vi "GUI_Plasma2_cap_pressure_cal.vi"() -> ()   [LabVIEW 2013]
uses:
  Shared/GUI_Template/GUI_master/tcp_new_data_event.ctl
  Shared/GUI_Template/GUI_master/tcp new data cluster.ctl
  <vilib>/Analysis/NI_AALBase.lvlib
  <vilib>/Analysis/NI_AALPro.lvlib
panel:
  in  "voltage::2":dbl=0.001 caption="voltage" min=0.0 max=30.0 format="%#.3f"
  in  "GUIdevice 2":string="P2-capHV"
  out "pressure::1":dbl=0.001 caption="Pressure" min=-100.0 max=500.0 format="%#.3f"
  in  "Tab Control":T1(tab)
  out "Pressure":dbl(graph)
  in  "points to save":T2(ring)
  in  "clear buffer":bool
  in  "send data":T2(ring)
  out "feed pressure":cluster{dbl[], dbl[]}(graph)
  out "cap pressure":cluster{dbl[], dbl[]}(graph)
  in  "combine plots":bool
  out "XY Graph 2":cluster{"ind":dbl[], "ini2":dbl[]}[](graph)=[{"ind"=[-2.02123979383, -1.9193278234999998, -1.81603094787, -1.7156190046100002, -1.6146447489499998, -1.51219345453, -1.4118886632300003, -1.3132607968099999, -1.20859797921, -1.10528298126, -0.99947359182, -0.89101754336, -0.7830056618400001, -0.6703321602099999, -0.560133506, -0.45195395803, -0.33700739742999997, -0.22552528281, -0.11709424518, -0.00137819706, 0.11140632129999999, 0.22448127726, 0.34074782323999997, 0.45065273575, 0.5650082886, 0.68208983815, 0.79504242345, 0.91265498684, 1.02879685929, 1.14707402107, 1.26927132994], "ini2"=[325.9, 334.1, 414.7, 495.2, 600.9, 746.4, 853.9, 1001.9, 1112.0, 1295.3, 1395.5, 1514.7, 1653.1, 1697.2, 1749.0, 1762.6, 1725.7, 1610.9, 1491.6, 1395.8, 1147.7, 1104.4, 888.0, 763.9, 613.5, 460.9, 375.1, 348.9, 338.1, 301.2, 290.0]}, {"ind"=[-2.02123979383, -2.02123979383, -2.02123979383, -1.9193278234999998, -1.9193278234999998, -1.9193278234999998, -1.81603094787, -1.81603094787, -1.81603094787, -1.7156190046100002, -1.7156190046100002, -1.7156190046100002, -1.6146447489499998, -1.6146447489499998, -1.6146447489499998, -1.51219345453, -1.51219345453, -1.51219345453, -1.4118886632300003, -1.4118886632300003, -1.4118886632300003, -1.3132607968099999, -1.3132607968099999, -1.3132607968099999, -1.20859797921, -1.20859797921, -1.20859797921, -1.10528298126, -1.10528298126, -1.10528298126, -0.99947359182, -0.99947359182, -0.99947359182, -0.89101754336, -0.89101754336, -0.89101754336, -0.7830056618400001, -0.7830056618400001, -0.7830056618400001, -0.6703321602099999, -0.6703321602099999, -0.6703321602099999, -0.560133506, -0.560133506, -0.560133506, -0.45195395803, -0.45195395803, -0.45195395803, -0.33700739742999997, -0.33700739742999997, -0.33700739742999997, -0.22552528281, -0.22552528281, -0.22552528281, -0.11709424518, -0.11709424518, -0.11709424518, -0.00137819706, -0.00137819706, -0.00137819706, 0.11140632129999999, 0.11140632129999999, 0.11140632129999999, 0.22448127726, 0.22448127726, 0.22448127726, 0.34074782323999997, 0.34074782323999997, 0.34074782323999997, 0.45065273575, 0.45065273575, 0.45065273575, 0.5650082886, 0.5650082886, 0.5650082886, 0.68208983815, 0.68208983815, 0.68208983815, 0.79504242345, 0.79504242345, 0.79504242345, 0.91265498684, 0.91265498684, 0.91265498684, 1.02879685929, 1.02879685929, 1.02879685929, 1.14707402107, 1.14707402107, 1.14707402107, 1.26927132994, 1.26927132994, 1.26927132994], "ini2"=[347.24088408040615, 304.5591159195938, nan, 345.14988687724906, 323.050113122751, nan, 451.6325210500327, 377.76747894996726, nan, 550.571071468372, 439.82892853162804, nan, 647.2044274341018, 554.5955725658981, nan, 805.5930926901291, 687.2069073098709, nan, 922.3502252248546, 785.4497747751453, nan, 1045.7974815779776, 958.0025184220223, nan, 1155.936823331284, 1068.063176668716, nan, 1360.6589235597473, 1229.9410764402526, nan, 1468.004789113854, 1322.995210886146, nan, 1570.967318321661, 1458.4326816783391, nan, 1710.4148225931904, 1595.7851774068095, nan, 1733.5311925974852, 1660.868807402515, nan, 1789.7376429798726, 1708.2623570201274, nan, 1800.3512325037946, 1724.8487674962053, nan, 1767.5623405408198, 1683.8376594591803, nan, 1653.6510883552169, 1568.1489116447833, nan, 1552.2083969246653, 1430.9916030753345, nan, 1464.0833963875716, 1327.5166036124283, nan, 1195.138966636675, 1100.2610333633252, nan, 1174.7928658001333, 1034.0071341998669, nan, 956.8896057310374, 819.1103942689626, nan, 863.6835991867734, 664.1164008132265, nan, 680.985389365238, 546.014610634762, nan, 522.2178422465906, 399.5821577534093, nan, 409.11127264109166, 341.0887273589084, nan, 373.0589642897943, 324.74103571020567, nan, 350.24221286806215, 325.9577871319379, nan, 316.5318839894733, 285.8681160105267, nan, 301.05541596785133, 278.94458403214867, nan]}] caption="output graph"
  out "slope":dbl
  out "intercept":dbl
  in  "GUIdevice 1":string="P2_PDR2000"
  in  "stop":bool
  out "tcp data event":T3
  out "error IO 2":errorcluster
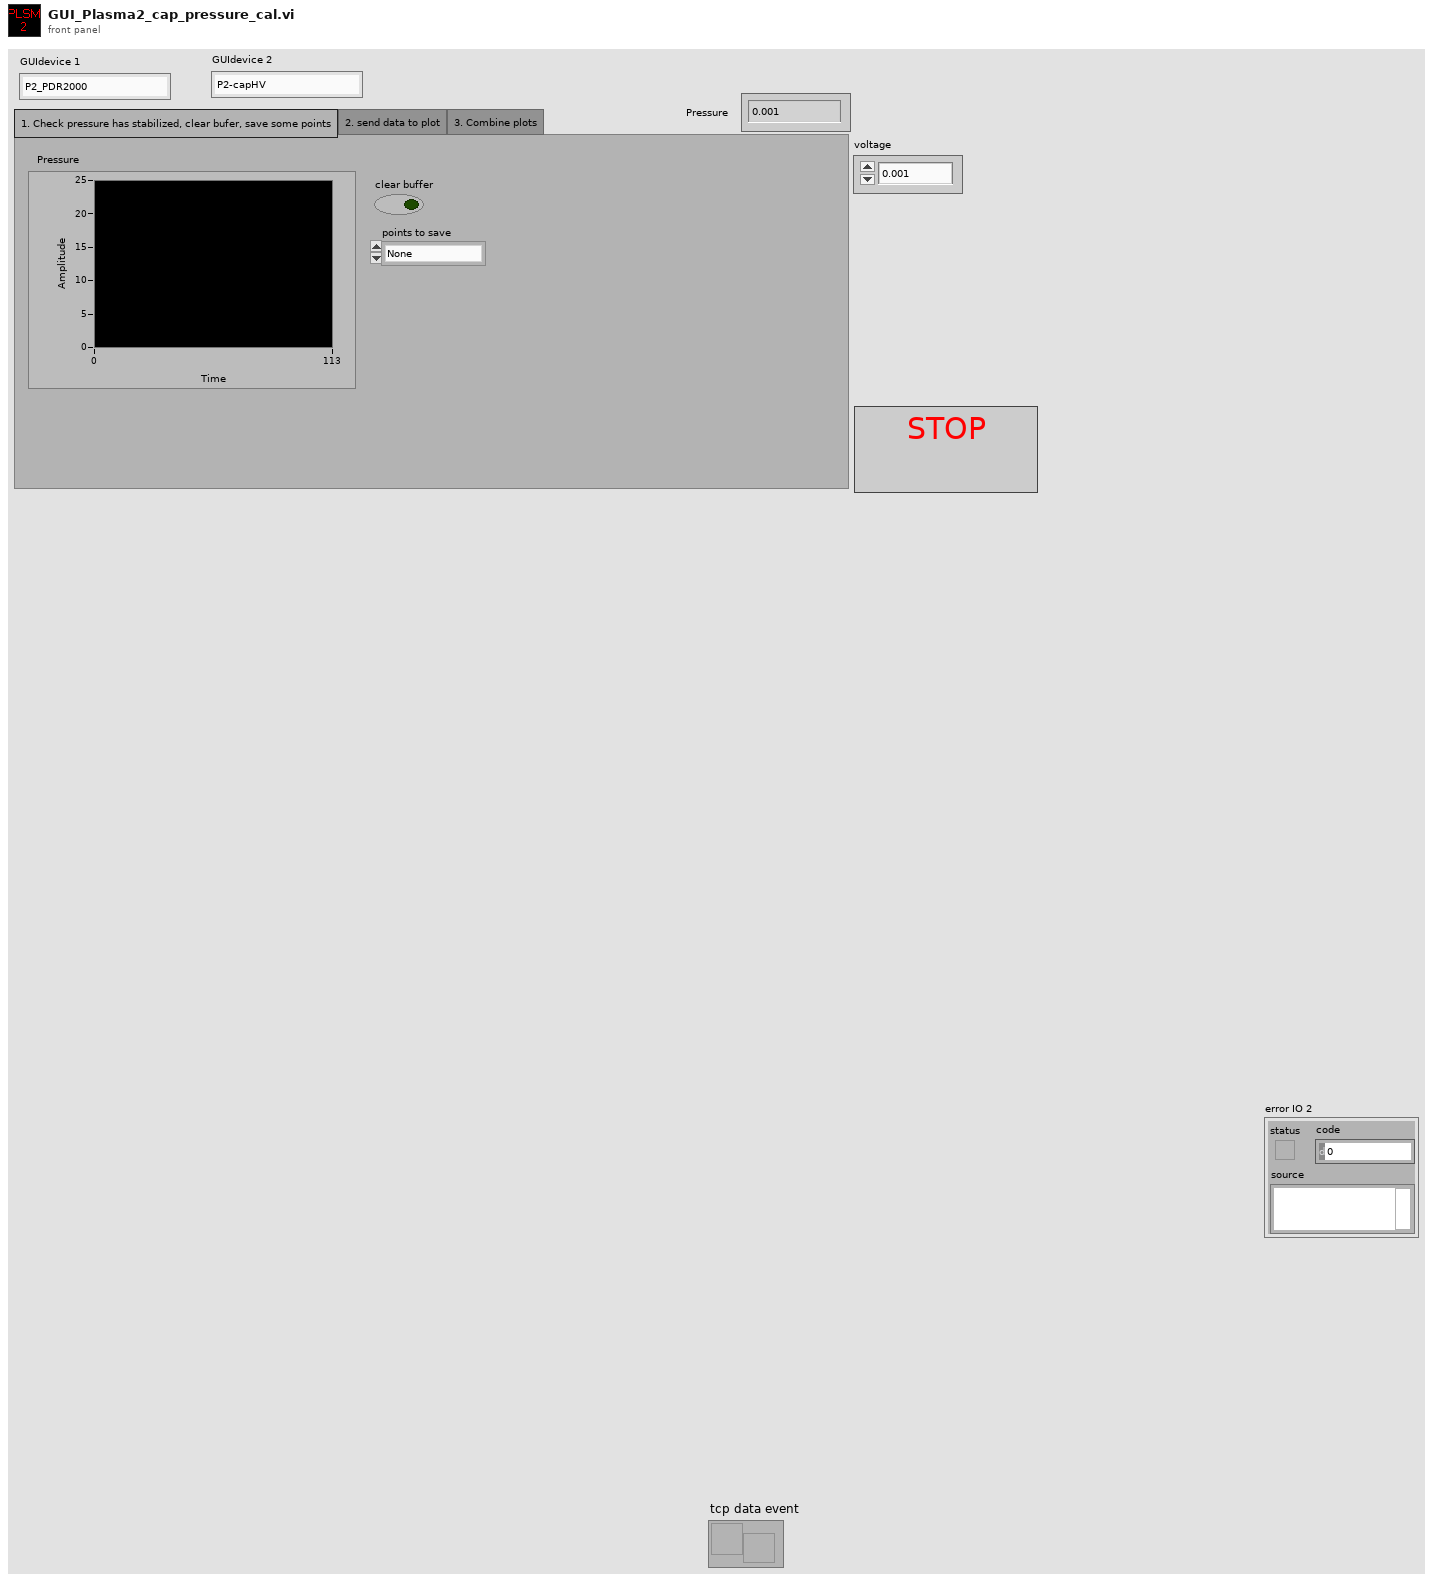
[diagram p1: front panel]
types:
  T1 = enum32{"1. Check pressure has stabilized, clear bufer, save some points", "2. send data to plot", "3. Combine plots"}
  T2 = enum16{"None", "Capillary pressure", "Feed pressure"}
  T3 = typedef "tcp_new_data_event.ctl" = refnum<user-event>
  T4 = typedef "tcp new data cluster.ctl" = cluster{"EventEnum":enum16{"new data", "connection status update"}, "Device name":string}
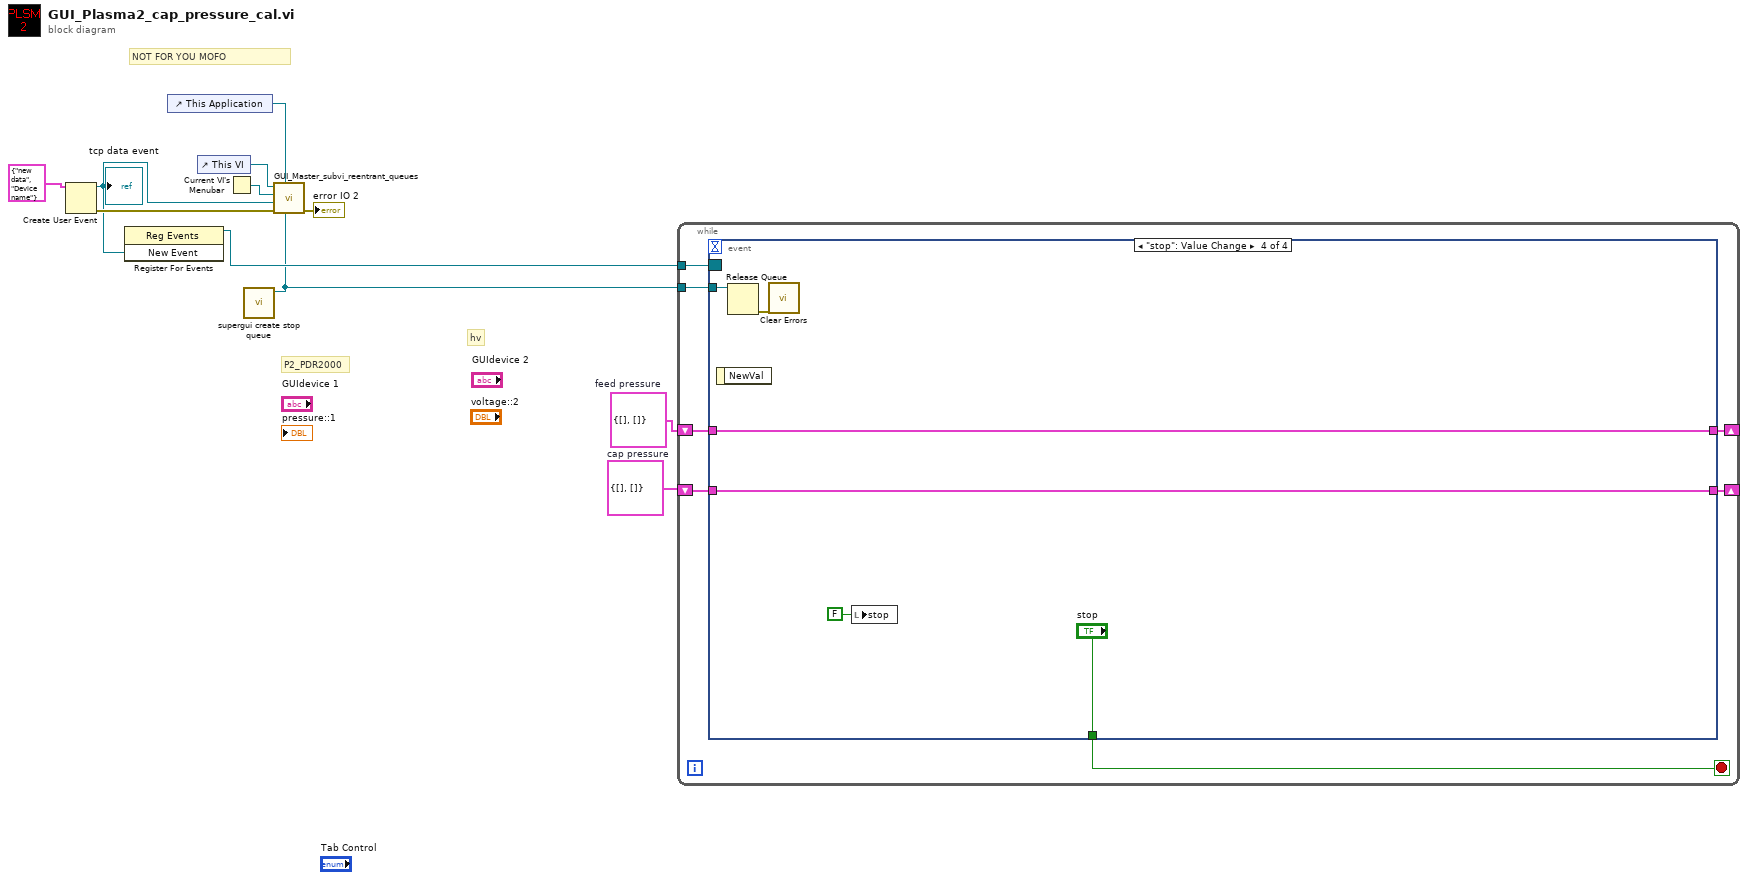
[diagram p0: block diagram]
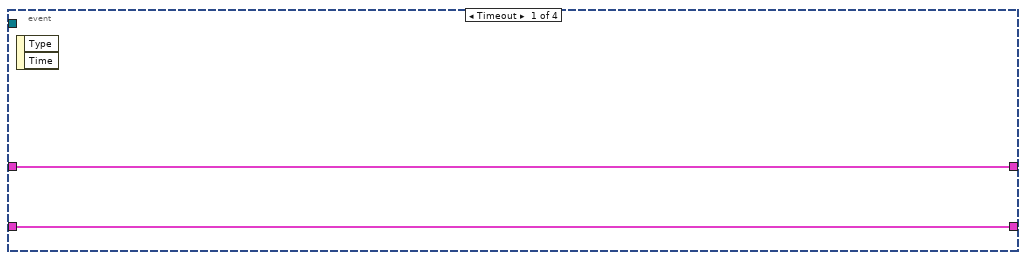
[diagram p2: hidden frame]
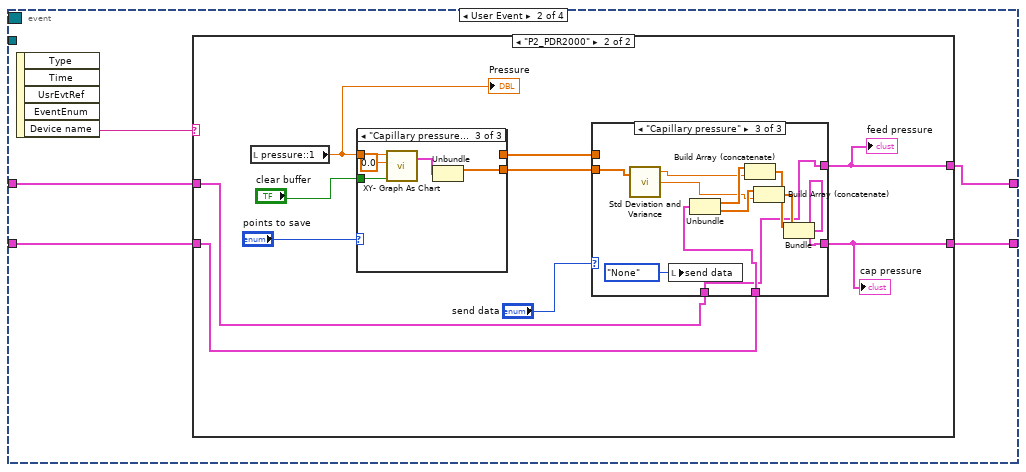
[diagram p3: hidden frame]
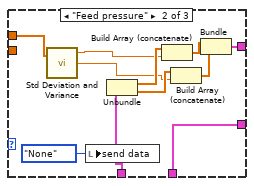
[diagram p6: hidden frame]
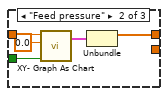
[diagram p8: hidden frame]
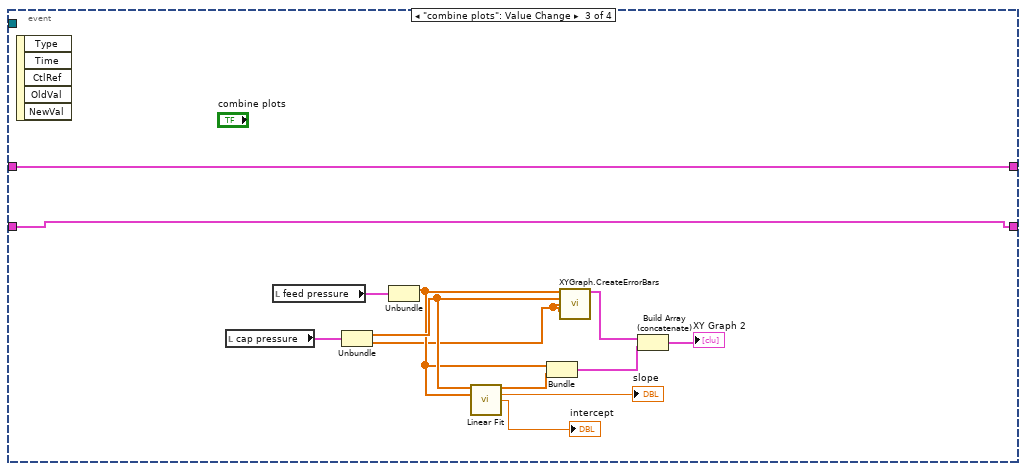
[diagram p9: hidden frame]
diagram:
  w2 = cluster{dbl[], dbl[]} {[], []}  # cap pressure
  w3 = cluster{dbl[], dbl[]} {[], []}  # feed pressure
  # "hv"
  # "P2_PDR2000"
  # "NOT FOR YOU MOFO"
  n1 = Create User Event(user event datatype=T4 {"EventEnum"=enum."new data", "Device name"="Device name"} ("New Event")) -> (user event=w6:refnum<user-event>, error out=w7:errorcluster)  [unwired: 1 in]
  "tcp data event" <- w6
  n2 = register-events(w6) -> (reference out=w4:refnum<event-registration>)  [unwired: 2 in, 1 out]
  n3 = control-ref of="This Application"() -> (w5:refnum<vi>)
  n4 = control-ref of="This VI"() -> (w10:refnum<vi>)
  n5 = Current VI's Menubar() -> (w9:refnum<k9>)
  n6 = call "supergui create stop queue.vi"() -> ("STOP Queue out"=w1:refnum<queue>)  [unwired: 11 in]
  n7 = call "GUI_Master_subvi_reentrant_queues.vi"("STOP Queue in"=w1, "This Application"=w5, "error in (no error)"=w7, "tcp data event"=w6, "Caller menu reference"=w9, "Caller VI ref"=w10) -> ("error out"=→"error IO 2":errorcluster)  [unwired: 5 in]
  n8 = while {
    tunnel: w4 -> [w17]
    shift-right: [w15] -> _
    shift-left: w3 -> [w16]
    shift-right: [w13] -> _
    shift-left: w2 -> [w14]
    tunnel: w1 -> [w12]
    stop <- w18 stop-if-true
    n9 = event shown="[3] \"stop\": Value Change" {
      selector: w17 -> [_ _ _ _]
      dyn-events: _ -> [_ _ _ _]
      timeout: _ -> [_ _ _ _]
      tunnel: [_ _ _ "stop"] -> w18
      tunnel: w16 -> [w20 w24 w74 w88]
      tunnel: [w20 w21 w74 w88] -> w15
      tunnel: w14 -> [w19 w23 w73 w87]
      tunnel: [w19 w22 w73 w87] -> w13
      tunnel: w12 -> [_ _ _ w86]
      event Timeout {
        n10 = event-data() -> ()  [unwired: 1 in, 2 out]
      }
      event User Event {
        n11 = event-data() -> ("Device name"=w25:string)  [unwired: 1 in, 4 out]
        n12 = case shown="\"P2_PDR2000\"" w25 {
          tunnel: w24 -> [w27 w30]
          tunnel: w23 -> [w26 w31]
          tunnel: [w26 w29] -> w22
          tunnel: [w27 w28] -> w21
          frame Default {
          }
          frame "P2_PDR2000" {
            n13 = local read "pressure::1"() -> (w36:dbl)
            "Pressure" <- w36
            n14 = case shown="\"Capillary pressure\"" "points to save" {
              tunnel: w36 -> [_ w66 w71]
              tunnel: "clear buffer" -> [_ w65 w70]
              tunnel: [_ w63 _] -> w32
              tunnel: [_ _ w68] -> w33
              frame "None", Default {
              }
              frame "Feed pressure" {
                n15 = call "XY- Graph As Chart.vi"("Wire in Stop To Clear Graph on Each Run"=w65, "Y-Value"=0.0, "X- Value"=w66) -> ("XY Graph"=w64:cluster{dbl[], dbl[]})  [unwired: 2 in]
                n16 = Unbundle(w64) -> (w63:dbl[])  [unwired: 1 out]
              }
              frame "Capillary pressure" {
                n17 = call "XY- Graph As Chart.vi"("Wire in Stop To Clear Graph on Each Run"=w70, "Y-Value"=0.0, "X- Value"=w71) -> ("XY Graph"=w69:cluster{dbl[], dbl[]})  [unwired: 2 in]
                n18 = Unbundle(w69) -> (w68:dbl[])  [unwired: 1 out]
              }
            }
            n19 = case shown="\"Capillary pressure\"" "send data" {
              tunnel: w33 -> [_ _ w51]
              tunnel: w32 -> [_ w49 _]
              tunnel: w31 -> [w38 w48 w53]
              tunnel: [w38 w48 w54] -> w29
              tunnel: w30 -> [w39 w47 w52]
              tunnel: [w39 w40 w52] -> w28
              frame "None", Default {
              }
              frame "Feed pressure" {
                n20 = call <vilib>:"Std Deviation and Variance.vi"("X"=w49) -> ("mean"=w44:dbl, "standard deviation"=w43:dbl)  [unwired: 1 in, 1 out]
                n21 = local write "send data"(T2."None" ("send data")) -> ()
                n22 = Unbundle(w47) -> (w46:dbl[], w45:dbl[])
                n23 = Build Array (concatenate)(w46, w44) -> (w42:dbl[])
                n24 = Build Array (concatenate)(w45, w43) -> (w41:dbl[])
                n25 = Bundle(w42, w41) -> (w40:cluster{dbl[], dbl[]})  [unwired: 1 in]
              }
              frame "Capillary pressure" {
                n26 = call <vilib>:"Std Deviation and Variance.vi"("X"=w51) -> ("mean"=w58:dbl, "standard deviation"=w57:dbl)  [unwired: 1 in, 1 out]
                n27 = local write "send data"(T2."None" ("send data")) -> ()
                n28 = Unbundle(w53) -> (w60:dbl[], w59:dbl[])
                n29 = Build Array (concatenate)(w60, w58) -> (w56:dbl[])
                n30 = Build Array (concatenate)(w59, w57) -> (w55:dbl[])
                n31 = Bundle(w56, w55) -> (w54:cluster{dbl[], dbl[]})  [unwired: 1 in]
              }
            }
            "feed pressure" <- w28
            "cap pressure" <- w29
          }
        }
      }
      event "combine plots": Value Change {
        n32 = event-data() -> ()  [unwired: 1 in, 5 out]
        n33 = local read "cap pressure"() -> (w84:cluster{dbl[], dbl[]})
        n34 = local read "feed pressure"() -> (w83:cluster{dbl[], dbl[]})
        n35 = Unbundle(w84) -> (w82:dbl[], w72:dbl[])
        n36 = Unbundle(w83) -> (w76:dbl[])  [unwired: 1 out]
        n37 = call <vilib>:"Linear Fit.vi"("Y"=w82, "X"=w76) -> ("Best Linear Fit"=w75:dbl[], "slope"=→"slope":dbl, "intercept"=→"intercept":dbl)  [unwired: 9 in, 2 out]
        n38 = Bundle(w76, "Best Linear Fit"=w75) -> (w77:cluster{dbl[], "Best Linear Fit":dbl[]})  [unwired: 1 in]
        n39 = call "XYGraph.CreateErrorBars.vi"("X"=w76, "Y"=w82, "error low"=w72, "error high"=w72) -> ("xy graph bin 2"=w79:cluster{"X":dbl[], "Y":dbl[]}[])  [unwired: 11 out]
        n40 = Build Array (concatenate)(w79, w77) -> (→"XY Graph 2":cluster{"X":dbl[], "Best Linear Fit":dbl[]}[])
      }
      event "stop": Value Change {
        n41 = event-data() -> ()  [unwired: 1 in, 1 out]
        n42 = Release Queue(queue=w86) -> (error out=w85:errorcluster)  [unwired: 2 in, 2 out]
        n43 = call <vilib>:"Clear Errors.vi"("error in (no error)"=w85) -> ()  [unwired: 6 in, 1 out]
        n44 = local write "stop"(FALSE ("stop")) -> ()
      }
    }
  }
